vi "Self test 9250.vi"(8 "error in (no error)":errorcluster, 11 "Accelerometer":T1) -> (0 "error out":errorcluster, 1 "accel self test":dbl[](array[numeric]), 2 "gyro self test":dbl[](array[numeric]), 3 "Accelerometer out":T1)   [LabVIEW 2013]
doc: "Use this template to build a VI to use as a subVI."
uses:
  9250registers.ctl
  <vilib>/ni845x/ni845x.llb/ni845xControl.ctl
  <vilib>/ni845x/ni845x.llb/ni845xSpiConfiguration.ctl
  AccelerometerSPI.ctl
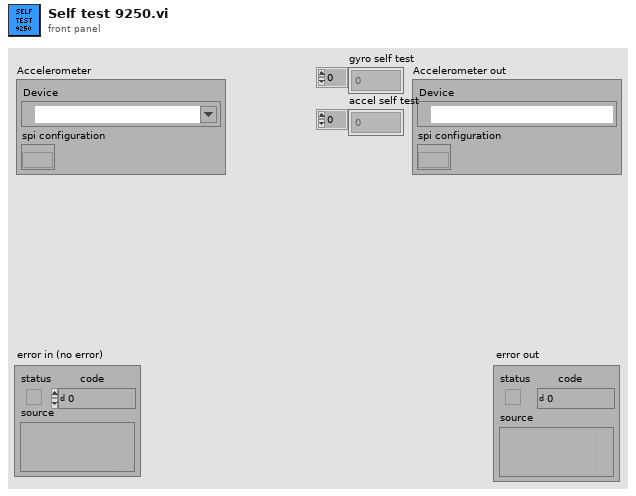
[diagram p1: front panel]
types:
  T1 = typedef "AccelerometerSPI.ctl" = cluster{"Device":T2, "spi configuration":T3}
  T2 = typedef "ni845xControl.ctl" = refnum<k21>
  T3 = typedef "ni845xSpiConfiguration.ctl" = refnum<k20>
  T4 = typedef "9250registers.ctl" = u8
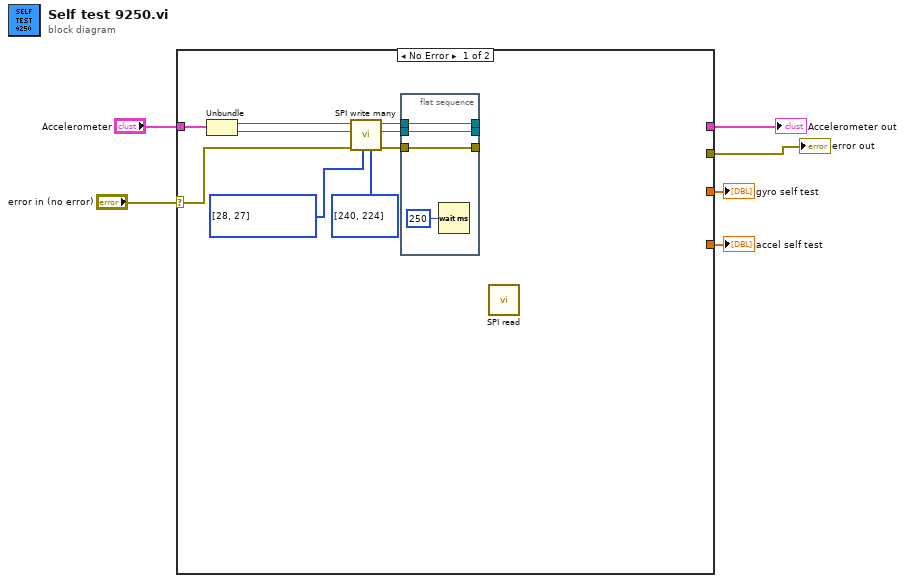
[diagram p0: block diagram]
diagram:
  n1 = case shown="No Error" "error in (no error)" {
    selector: "error in (no error)" -> [w10 w22]
    tunnel: [_ w22] -> w5
    tunnel: "Accelerometer" -> [w15 w21]
    tunnel: [_ w21] -> w3
    tunnel: [_ _] -> w2
    tunnel: [w16 _] -> w1
    frame No Error {
      w11 = T4[] [28, 27] items=["SELF_TEST_X_GYRO"=0, "SELF_TEST_Y_GYRO"=1, "SELF_TEST_Z_GYRO"=2, "SELF_TEST_X_ACCEL"=13, "SELF_TEST_Y_ACCEL"=14, "SELF_TEST_Z_ACCEL"=15, "XG_OFFSET"=19, "YG_OFFSET"=21, "ZG_OFFSET"=23, "SMPLRT_DIV"=25, "CONFIG"=26, "GYRO_CONFIG"=27, "ACCEL_CONFIG"=28, "ACCEL_CONFIG2"=29, "FIFO_EN"=35, "I2C_MST_CTRL"=36, "I2C_SLV0_ADDR"=37, "I2C_SLV0_REG"=38, "I2C_SLV0_CTRL"=39, "I2C_MST_STATUS"=54, "INT_ENABLE"=56, "INT_STATUS"=58, "ACCEL_XOUT"=59, "ACCEL_YOUT"=61, "ACCEL_ZOUT"=63, "TEMP_OUT"=65, "GYRO_XOUT"=67, "GYRO_YOUT"=69, "GYRO_ZOUT"=71, "EXT_SENS_DATA_00"=73, "I2C_SLV0_D0"=99, "USER_CTRL"=106, "PWR_MGMT_1"=107, "PWR_MGMT_2"=108, "WHO_AM_I"=117, "XA_OFFSET"=119, "YA_OFFSET"=122, "ZA_OFFSET"=125] ("addresses")
      n2 = Unbundle(w15) -> ("Device"=w13:T2, "spi configuration"=w14:T3)
      n3 = call "SPI write many.vi"("values"=u8[] [240, 224], "addresses"=w11, "error in (no error)"=w10, "spi configuration in"=w14, "Device ref in"=w13) -> ("error out"=w7:errorcluster, "spi configuration out"=w8:T3, "Device ref out"=w9:T2)  [unwired: 4 in]
      n4 = flat-sequence {
        tunnel: w9 -> [w19]
        tunnel: w8 -> [w18]
        tunnel: w7 -> [w17]
        tunnel: [w19] -> _
        tunnel: [w18] -> _
        tunnel: [w17] -> _
        frame #0 {
          n5 = Wait (ms)(milliseconds to wait=u32 250) -> ()  [unwired: 1 out]
        }
      }
      n6 = call "SPI read.vi"() -> ()  [unwired: 8 in, 4 out]
    }
    frame Error {
    }
  }
  "error out" <- w5
  "Accelerometer out" <- w3
  "gyro self test" <- w2
  "accel self test" <- w1
